vi "formatString.vi"(9 "Value":string, 11 "StringFormatter":refnum<class "StringFormatter.lvclass">) -> (1 "Formatted Value":string)   [LabVIEW 2013, in "OpenStringFormatter.lvlib" / "StringFormatter.lvclass"]
uses:
  StringFormatter.lvclass
  StringFormatter.lvclass/StringFormatter.ctl
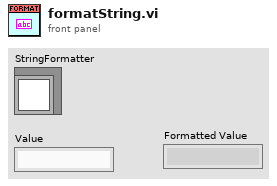
[diagram p1: front panel]
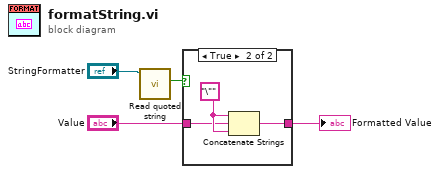
[diagram p0: block diagram]
diagram:
  n1 = call "Read quoted string.vi"("StringFormatter in"="StringFormatter") -> ("quoted string"=w4:bool)  [unwired: 9 in, 1 out]
  n2 = case shown="True" w4 {
    tunnel: [w5 w7] -> w1
    tunnel: "Value" -> [w5 w6]
    frame False {
    }
    frame True {
      w8 = "\"" ("string")
      n3 = Concatenate Strings(w8, w6, w8) -> (w7:string)
    }
  }
  "Formatted Value" <- w1
